vi "MakeSteps.vi"(0 "Axis":T2 items=["Axis 1", "Axis 2", "Axis 3"], 1 "Number":i32=-2147483648, 5 "error in":T1) -> (14 "Output Cluster":cluster{"Axis":i32, "Number":i32}, 19 "error out":T1)   [LabVIEW 2016]
doc: "This VI initiates a 'number' of steps for the specified axis, which is of course a required input and runs from 0 to 2."
uses:
  Controls/Coarse-Axis_Selection.ctl
  Controls/Error_Out.ctl
  Files_ASC500/DLL/ASC500_RemoteControlV27.dll
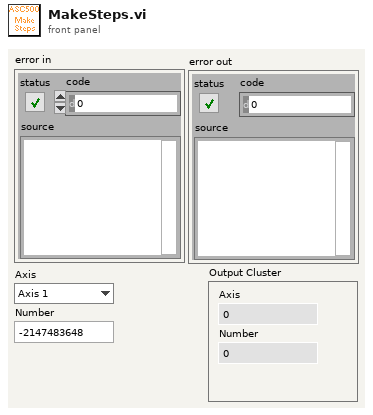
[diagram p1: front panel]
types:
  T1 = typedef "Error_Out.ctl" = errorcluster
  T2 = typedef "Coarse-Axis_Selection.ctl" = u16
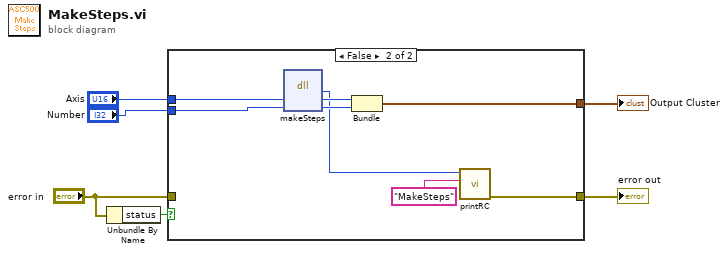
[diagram p0: block diagram]
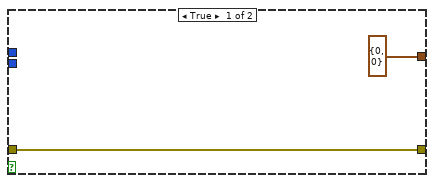
[diagram p2: hidden frame]
diagram:
  n1 = Unbundle By Name("error in") -> ("status"=w6:bool)
  n2 = case shown="False" w6 {
    tunnel: [w7 w10] -> w5
    tunnel: "Number" -> [_ w14]
    tunnel: "Axis" -> [_ w13]
    tunnel: [cluster{"Axis":i32, "Number":i32} {"Axis"=0, "Number"=0} w12] -> w2
    tunnel: "error in" -> [w7 _]
    frame True {
    }
    frame False {
      n3 = dll-call lib="G:/SCMOperations/Share/ELE/Produkt Information/ASC500/04 Remote Control/02 development versions/2018Nov06/Files_ASC500/DLL/ASC500_RemoteControlV27.dll" fn="makeSteps"("Axis"=w13, "Number"=w14) -> ("return type"=w11:i32, "Axis"=w16:i32, "Number"=w15:i32)  [unwired: 3 in, 2 out]
      n4 = Bundle("Axis"=w16, "Number"=w15) -> (w12:cluster{"Axis":i32, "Number":i32})  [unwired: 1 in]
      n5 = call "printRC.vi"("additional information"="MakeSteps", "RC"=w11) -> ("error out"=w10:T1)  [unwired: 9 in]
    }
  }
  "error out" <- w5
  "Output Cluster" <- w2
